vi "EMS Get Measurement Status.vi"(4 "Measurement/Error":string, 6 "Status":T1, 8 "error in (no error)":errorcluster, 9 "Measurement Name":string, 10 "IED Name":string, 11 "Master Controller in":refnum<class "Master Controller.lvclass">) -> (0 "error out":errorcluster, 3 "Master Controller out":refnum<class "Master Controller.lvclass">)   [LabVIEW 2015, in "Master Controller Core.lvlib" / "Master Controller.lvclass"]
uses:
  Master Controller.lvclass
  SCADA Core/SCADA Abstract Messages/IED Measurement Status Msg/IED Measurement Status.ctl
  Communications/SCADA Communcations Actor/SCADA Communications/Controls/EMS Message Cluster.ctl
  Master Controller.lvclass/Master Controller.ctl
  Communications/SCADA Communcations Actor/SCADA Communications Messages/Transmit EMS Message Msg/Transmit EMS Message Msg.lvclass/Transmit EMS Message Msg.ctl
  <vilib>/ActorFramework/Message Enqueuer/Message Enqueuer.lvclass/Message Enqueuer.ctl
  <vilib>/ActorFramework/Message Enqueuer/Enqueue.vi
  <vilib>/ActorFramework/Message Priority Queue/Priority Enqueue.vi
  Communications/SCADA Communcations Actor/SCADA Communications Messages/Transmit EMS Message Msg/Transmit EMS Message Msg.lvclass
  Utilities/Message Strings.llb/Message String Utilities.lvlib
  Communications/SCADA Communcations Actor/SCADA Communications/SCADA Communications.lvclass
  SCADA Core/SCADA Abstract Messages/IED Measurement Status Msg/IED Measurement Status Msg.lvclass
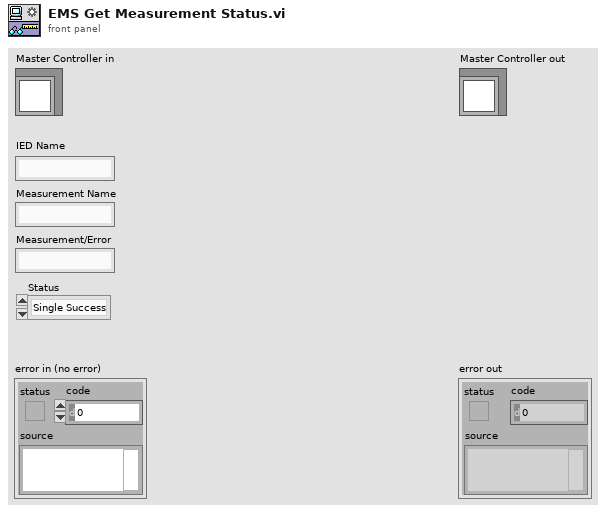
[diagram p1: front panel]
types:
  T1 = typedef "SCADA Core.lvlib/IED Measurement Status Msg.lvclass/IED Measurement Status.ctl" = enum16{"Single Success", "Single Failure", "Multiple Success", "Multiple Failure"}
  T2 = typedef "SCADA Communcations Actor.lvlib/SCADA Communications.lvclass/EMS Message Cluster.ctl" = cluster{"Name":string, "Content":string}
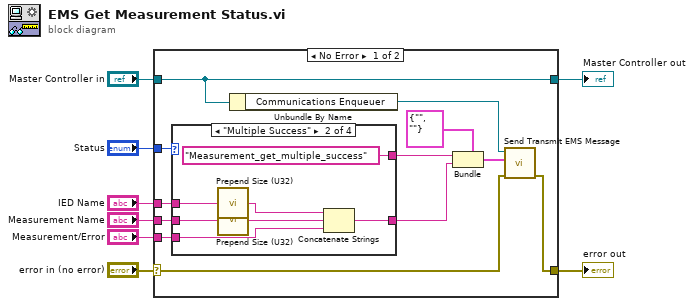
[diagram p0: block diagram]
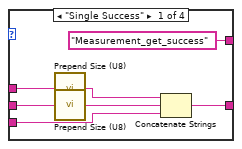
[diagram p2: hidden frame]
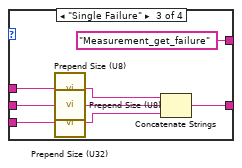
[diagram p3: hidden frame]
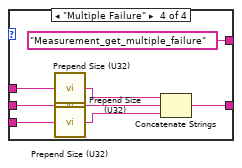
[diagram p4: hidden frame]
diagram:
  n1 = case shown="No Error" "error in (no error)" {
    selector: "error in (no error)" -> [w15 w52]
    tunnel: [w14 w52] -> w7
    tunnel: [w16 w51] -> w5
    tunnel: "Master Controller in" -> [w16 w51]
    tunnel: "Status" -> [w13 _]
    tunnel: "IED Name" -> [w12 _]
    tunnel: "Measurement Name" -> [w11 _]
    tunnel: "Measurement/Error" -> [w10 _]
    frame No Error {
      n2 = case shown="\"Multiple Success\"" w13 {
        tunnel: ["Measurement_get_success" ("Name") "Measurement_get_multiple_success" ("Name") "Measurement_get_failure" ("Name") "Measurement_get_multiple_failure" ("Name")] -> w20
        tunnel: w12 -> [w24 w31 w37 w49]
        tunnel: w11 -> [w23 w30 w36 w48]
        tunnel: w10 -> [w21 w28 w35 w47]
        tunnel: [w22 w29 w38 w43] -> w9
        frame "Single Success" {
          n3 = call "Prepend Size (U8).vi"("String in"=w24) -> ("String out"=w25:string)
          n4 = call "Prepend Size (U8).vi"("String in"=w23) -> ("String out"=w26:string)
          n5 = Concatenate Strings(w25, w26, w21) -> (w22:string)
        }
        frame "Multiple Success" {
          n6 = call "Prepend Size (U32).vi"("String in"=w31) -> ("String out"=w32:string)
          n7 = call "Prepend Size (U32).vi"("String in"=w30) -> ("String out"=w33:string)
          n8 = Concatenate Strings(w32, w33, w28) -> (w29:string)
        }
        frame "Single Failure" {
          n9 = call "Prepend Size (U8).vi"("String in"=w37) -> ("String out"=w40:string)
          n10 = call "Prepend Size (U8).vi"("String in"=w36) -> ("String out"=w41:string)
          n11 = call "Prepend Size (U32).vi"("String in"=w35) -> ("String out"=w39:string)
          n12 = Concatenate Strings(w40, w41, w39) -> (w38:string)
        }
        frame "Multiple Failure" {
          n13 = call "Prepend Size (U32).vi"("String in"=w49) -> ("String out"=w44:string)
          n14 = call "Prepend Size (U32).vi"("String in"=w48) -> ("String out"=w45:string)
          n15 = call "Prepend Size (U32).vi"("String in"=w47) -> ("String out"=w46:string)
          n16 = Concatenate Strings(w44, w45, w46) -> (w43:string)
        }
      }
      n17 = Unbundle By Name(w16) -> ("Communications Enqueuer"=w18:refnum<class "Message Enqueuer.lvclass">)
      n18 = Bundle(cluster=T2 {"Name"="", "Content"=""} ("Message"), "Name"=w20, "Content"=w9) -> (w19:T2)
      n19 = call "Send Transmit EMS Message.vi"("error in (no error)"=w15, "Message"=w19, "Message Enqueuer"=w18) -> ("error out"=w14:errorcluster)  [unwired: 7 in, 1 out]
    }
    frame Error {
    }
  }
  "error out" <- w7
  "Master Controller out" <- w5
